vi "Initialize.vi"(8 "error in (no error)":errorcluster, 11 "S4ACS_GUI in":refnum<class "GuiderSetup.lvclass">) -> (0 "error out":errorcluster, 3 "S4ACS_GUI out":refnum<class "GuiderSetup.lvclass">)   [LabVIEW 2018, in "GuiderSetup.lvclass"]
uses:
  GuiderSetup.lvclass
  C:/Users/devstaff/sparc4/s4gui/Versao ZeroMQ REQ-REP/SPARC4_GUI -v1.0.8 - reconhecimento do ACK do ACS/S4GUI/S4GUI.lvclass
  S4GUI/S4GUI.lvclass/S4GUI.ctl
  GuiderSetup.lvclass/GuiderSetup.ctl
  Instrument/Instrument.lvclass
  Client_s4gui/Client_s4gui.lvclass
  PublisherGS/PublisherGS.lvclass
  AG/AG.lvclass
  S4GUI/S4GUI.lvclass
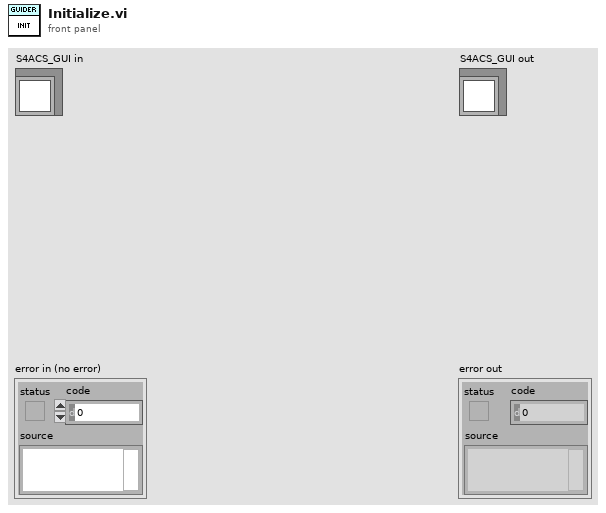
[diagram p1: front panel]
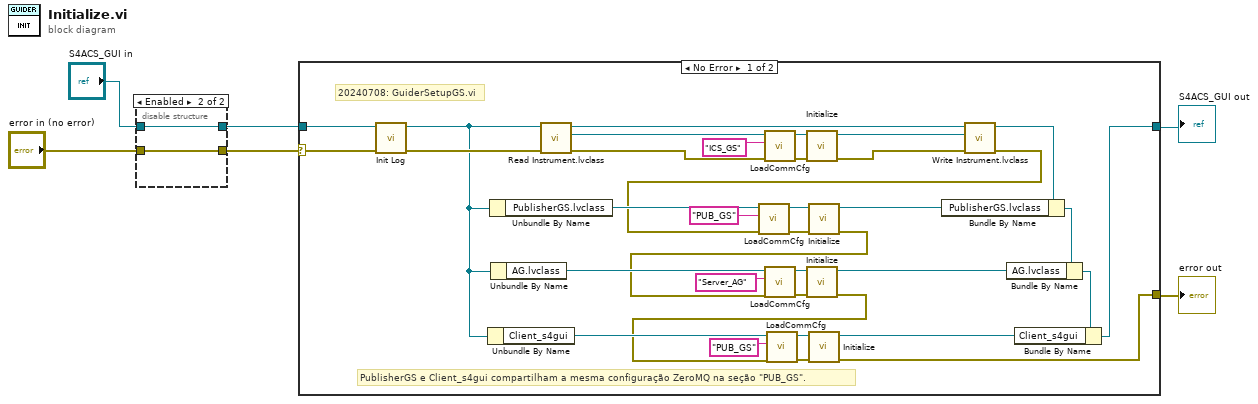
[diagram p0: block diagram]
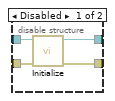
[diagram p2: hidden frame]
diagram:
  n1 = disable-structure shown="Enabled" {
    disable-tunnel: "error in (no error)" -> [w10 w11]
    disable-tunnel: "S4ACS_GUI in" -> [w9 w12]
    disable-tunnel: [w8 w12] -> w4
    disable-tunnel: [w7 w11] -> w3
    frame Disabled {
      n2 = call-parent "Initialize.vi"("error in (no error)"=w10, "S4ACS_GUI in"=w9) -> ("error out"=w7:errorcluster, "S4ACS_GUI out"=w8:refnum<class "GuiderSetup.lvclass">)  [unwired: 8 in]
    }
    frame Enabled {
    }
  }
  n3 = case shown="No Error" w3 {
    selector: w3 -> [w24 w48]
    tunnel: w4 -> [w25 w49]
    tunnel: [w13 w48] -> w1
    tunnel: [w15 w49] -> w2
    frame No Error {
      # "PublisherGS e Client_s4gui compartilham a mesma configuração ZeroMQ na seção \"PUB_GS\"."
      # "20240708: GuiderSetupGS.vi"
      n4 = call-dynamic "Init Log.vi"("error in (no error)"=w24, "GuiderSetup in"=w25) -> ("error out"=w23:errorcluster, "GuiderSetup out"=w17:refnum<class "GuiderSetup.lvclass">)  [unwired: 8 in]
      n5 = Unbundle By Name(w17) -> ("Client_s4gui"=w21:refnum<class "Client_s4gui.lvclass">)
      n6 = Unbundle By Name(w17) -> ("PublisherGS.lvclass"=w29:refnum<class "PublisherGS.lvclass">)
      n7 = Unbundle By Name(w17) -> ("AG.lvclass"=w42:refnum<class "AG.lvclass">)
      n8 = call "Read Instrument.lvclass.vi"("error in (no error)"=w23, "S4ACS_GUI in"=w17) -> ("error out"=w45:errorcluster, "Instrument.lvclass"=w46:refnum<class "Instrument.lvclass">, "S4ACS_GUI out"=w36:refnum<class "GuiderSetup.lvclass">)  [unwired: 7 in]
      n9 = call-dynamic "LoadCommCfg.vi"("error in (no error)"=w45, "section (server name)"="ICS_GS", "Server in"=w46) -> ("error out"=w44:errorcluster, "Server out"=w43:refnum<class "Instrument.lvclass">)  [unwired: 7 in]
      n10 = call-dynamic "Initialize.vi"("error in (no error)"=w44, "Instrument in"=w43) -> ("error out"=w35:errorcluster, "Instrument out"=w37:refnum<class "Instrument.lvclass">)  [unwired: 8 in]
      n11 = call "Write Instrument.lvclass.vi"("error in (no error)"=w35, "Instrument.lvclass"=w37, "S4ACS_GUI in"=w36) -> ("error out"=w27:errorcluster, "S4ACS_GUI out"=w31:refnum<class "GuiderSetup.lvclass">)  [unwired: 7 in]
      n12 = call-dynamic "LoadCommCfg.vi"("error in (no error)"=w27, "section (server name)"="PUB_GS", "Client in"=w29) -> ("error out"=w33:errorcluster, "Client out"=w32:refnum<class "PublisherGS.lvclass">)  [unwired: 7 in]
      n13 = call-dynamic "Initialize.vi"("error in (no error)"=w33, "Client in"=w32) -> ("error out"=w26:errorcluster, "Client out"=w28:refnum<class "PublisherGS.lvclass">)  [unwired: 8 in]
      n14 = call-dynamic "LoadCommCfg.vi"("error in (no error)"=w26, "section (server name)"="Server_AG", "Client in"=w42) -> ("error out"=w40:errorcluster, "Client out"=w41:refnum<class "AG.lvclass">)  [unwired: 7 in]
      n15 = call-dynamic "Initialize.vi"("error in (no error)"=w40, "AG in"=w41) -> ("error out"=w16:errorcluster, "AG out"=w47:refnum<class "AG.lvclass">)  [unwired: 8 in]
      n16 = call-dynamic "LoadCommCfg.vi"("error in (no error)"=w16, "section (server name)"="PUB_GS", "Client in"=w21) -> ("error out"=w19:errorcluster, "Client out"=w20:refnum<class "Client_s4gui.lvclass">)  [unwired: 7 in]
      n17 = call-dynamic "Initialize.vi"("error in (no error)"=w19, "Client in"=w20) -> ("error out"=w13:errorcluster, "Client out"=w22:refnum<class "Client_s4gui.lvclass">)  [unwired: 8 in]
      n18 = Bundle By Name(cluster=w31, "PublisherGS.lvclass"=w28) -> (w30:refnum<class "GuiderSetup.lvclass">)
      n19 = Bundle By Name(cluster=w30, "AG.lvclass"=w47) -> (w14:refnum<class "GuiderSetup.lvclass">)
      n20 = Bundle By Name(cluster=w14, "Client_s4gui"=w22) -> (w15:refnum<class "GuiderSetup.lvclass">)
    }
    frame Error {
    }
  }
  "error out" <- w1
  "S4ACS_GUI out" <- w2
